vi "LooadAxis.vi"(8 "error in (no error)":errorcluster, 11 "MPC_VirbVision in":refnum<class "MPC_VirbVision.lvclass">) -> (0 "error out":errorcluster, 2 "This VI":refnum<vi>, 3 "MPC_VirbVision out":refnum<class "MPC_VirbVision.lvclass">)   [LabVIEW 2019, in "MPC_VirbVision.lvclass"]
uses:
  MPC_VirbVision.lvclass
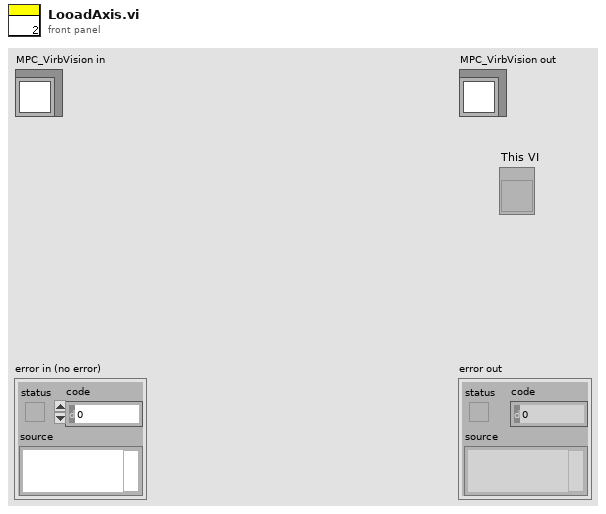
[diagram p1: front panel]
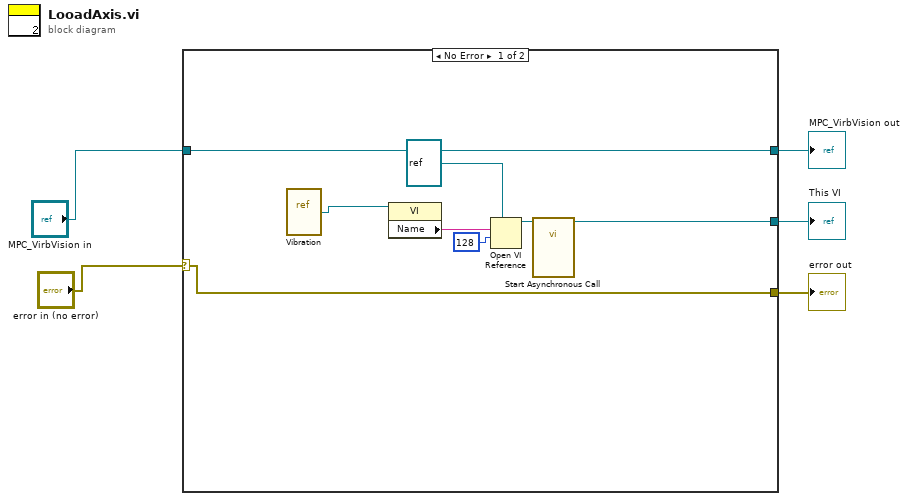
[diagram p0: block diagram]
diagram:
  n1 = case shown="No Error" "error in (no error)" {
    selector: "error in (no error)" -> [w13 w14]
    tunnel: [w13 w14] -> w4
    tunnel: "MPC_VirbVision in" -> [w12 w15]
    tunnel: [w12 w15] -> w2
    tunnel: [w7 _] -> w1
    frame No Error {
      n2 = vi-ref "Vibration.vi"() -> (w6:refnum<vi>)
      n3 = property class="VI"(reference=w6) -> ("Name"=w8:string)  [unwired: 1 in, 2 out]
      n4 = Open VI Reference(type specifier VI Refnum (for type only)=refnum<vi> refnum, vi path=w8, options=128) -> (vi reference=w11:refnum<vi>)  [unwired: 3 in, 1 out]
      n5 = call-by-ref "Start Asynchronous Call"(reference=w11) -> (reference out=w7:refnum<vi>)  [unwired: 13 in, 1 out]
    }
    frame Error {
    }
  }
  "error out" <- w4
  "MPC_VirbVision out" <- w2
  "This VI" <- w1
